vi "Create References.vi"(8 "error in (no error)":errorcluster, 11 "Engine in":refnum<class "Engine.lvclass">) -> (0 "error out":errorcluster, 3 "Engine out":refnum<class "Engine.lvclass">)   [LabVIEW 2023, in "Engine.lvlib" / "Engine.lvclass"]
doc: "Create reference is only called at the engine layer during the pre-launch init override. \n\nConditional operation as a function of <b>IsRoot</b>\n\n<b>IsRoot == TRUE</b>\nThis is the root actor, there is no expected caller reference, the event queues are uninitialized, and the data value references are uninitialized. So this option calls \n<b>Read Self Queue</b>\n<b>Create Report Queue</b>\n<b>Create Events</b>\n<b>Create DVRs</b>\n\n<b>IsRoot == FALSE</b>\nThis is a Nested Actor, and needs access to the caller enqueuer, so this condition calls:\n<b>Read Self Queue</b>\n<b>Read Caller Queue</b>"
uses:
  Library/Engine.lvclass
  C:/Users/Public/Documents/Development/builds/Framework/Actor Framework.lvlibp/1abvi3w/vi.lib/ActorFramework/Actor/Actor.lvclass
  Library/Engine.lvclass/Engine.ctl
  builds/Framework/Actor Framework.lvlibp/1abvi3w/vi.lib/ActorFramework/Actor/Actor.lvclass
  builds/Tools/QDMH.lvlibp/Library/QDMH.lvclass
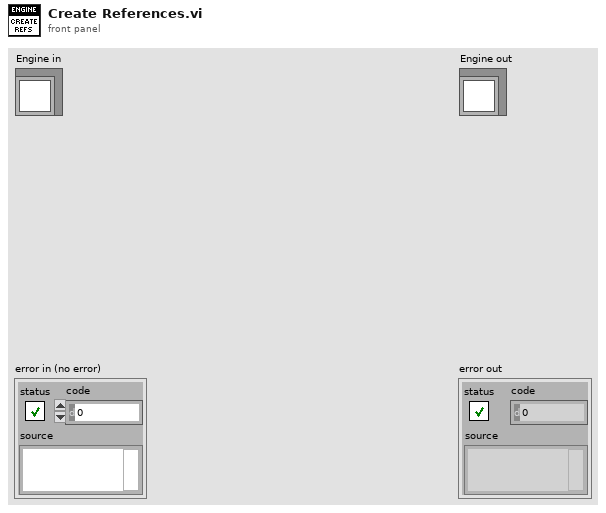
[diagram p1: front panel]
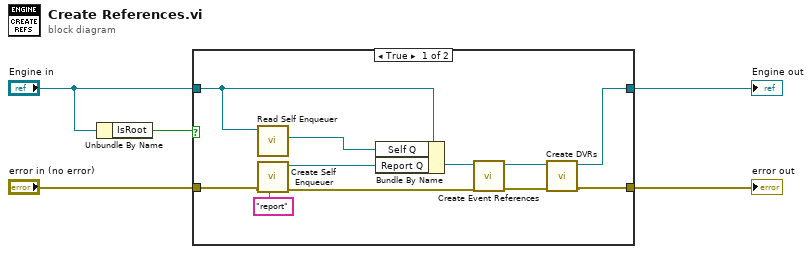
[diagram p0: block diagram]
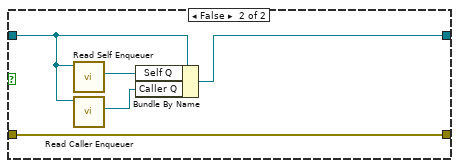
[diagram p2: hidden frame]
diagram:
  n1 = Unbundle By Name("Engine in") -> ("IsRoot"=w5:bool)
  n2 = case shown="True" w5 {
    tunnel: "Engine in" -> [w16 w19]
    tunnel: [w12 w20] -> w3
    tunnel: [w7 w17] -> w2
    tunnel: "error in (no error)" -> [w6 w17]
    frame True {
      n3 = call "Read Self Enqueuer.vi"("Actor"=w16) -> ("Self Enqueuer"=w15:refnum<class "Message Enqueuer.lvclass">)  [unwired: 10 in]
      n4 = call "Create Self Enqueuer.vi"("Name"="report", "error in (no error)"=w6) -> ("error out"=w9:errorcluster, "QDMH out"=w10:refnum<class "QDMH.lvclass">)  [unwired: 8 in]
      n5 = Bundle By Name(cluster=w16, "Self Q"=w15, "Report Q"=w10) -> (w13:refnum<class "Engine.lvclass">)
      n6 = call "Create Event References.vi"("error in (no error)"=w9, "Engine in"=w13) -> ("error out"=w8:errorcluster, "Engine out"=w14:refnum<class "Engine.lvclass">)  [unwired: 8 in]
      n7 = call "Create DVRs.vi"("error in (no error)"=w8, "Engine in"=w14) -> ("error out"=w7:errorcluster, "Engine out"=w12:refnum<class "Engine.lvclass">)  [unwired: 8 in]
    }
    frame False {
      n8 = call "Read Self Enqueuer.vi"("Actor"=w19) -> ("Self Enqueuer"=w21:refnum<class "Message Enqueuer.lvclass">)  [unwired: 10 in]
      n9 = call "Read Caller Enqueuer.vi"("Actor"=w19) -> ("Caller Enqueuer"=w18:refnum<class "Message Enqueuer.lvclass">)  [unwired: 10 in]
      n10 = Bundle By Name(cluster=w19, "Self Q"=w21, "Caller Q"=w18) -> (w20:refnum<class "Engine.lvclass">)
    }
  }
  "error out" <- w2
  "Engine out" <- w3
